vi "SIM_String Pot2016.vi"() -> (1 "Distance (in)":dbl=66.07442868832806 format="%.2f")   [LabVIEW 2016]
panel:
  in  "increment":dbl=1.0 format="%.2f"
  in  "sim_low":dbl format="%.2f"
  in  "sim_high":dbl=100.0 format="%.2f"
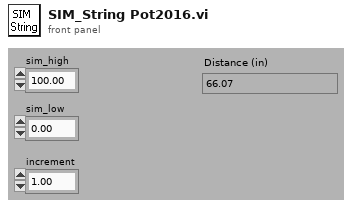
[diagram p1: front panel]
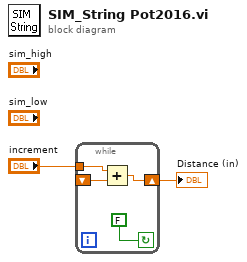
[diagram p0: block diagram]
diagram:
  n1 = while {
    tunnel: "increment" -> [w3]
    shift-left: _ -> [w5]
    shift-right: [w4] -> w1
    stop <- FALSE continue-if-true
    n2 = Add(x=w3, y=w5) -> (x+y=w4:dbl)
  }
  "Distance (in)" <- w1
